vi "SimulationLoop.vi"(0 "connection ID":refnum<k5>, 7 "Cluster":T1, 11 "error in (no error)":errorcluster, 12 "Stop Simulation":bool, 13 "filter":bool=TRUE caption="Filter") -> (4 "connection ID out":refnum<k5>, 6 "Velocity":cluster{"vx":dbl, "vy":dbl, "vy":dbl}, 8 "Acceleration":cluster{"ax":dbl, "ay":dbl, "az":dbl}, 10 "Speed":i32, 14 "Simulation Ended":bool, 15 "error out":errorcluster)   [LabVIEW 2019]
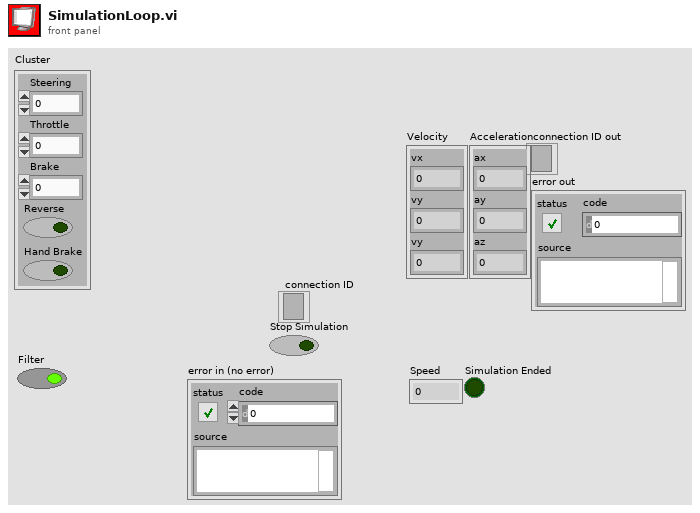
[diagram p1: front panel]
types:
  T1 = cluster{"Steering":i32, "Throttle":i32, "Brake":i32, "Reverse":bool, "Hand Brake":bool}
  T2 = cluster{"Filtered x":dbl, "Filtered x":dbl, "Filtered x":dbl}
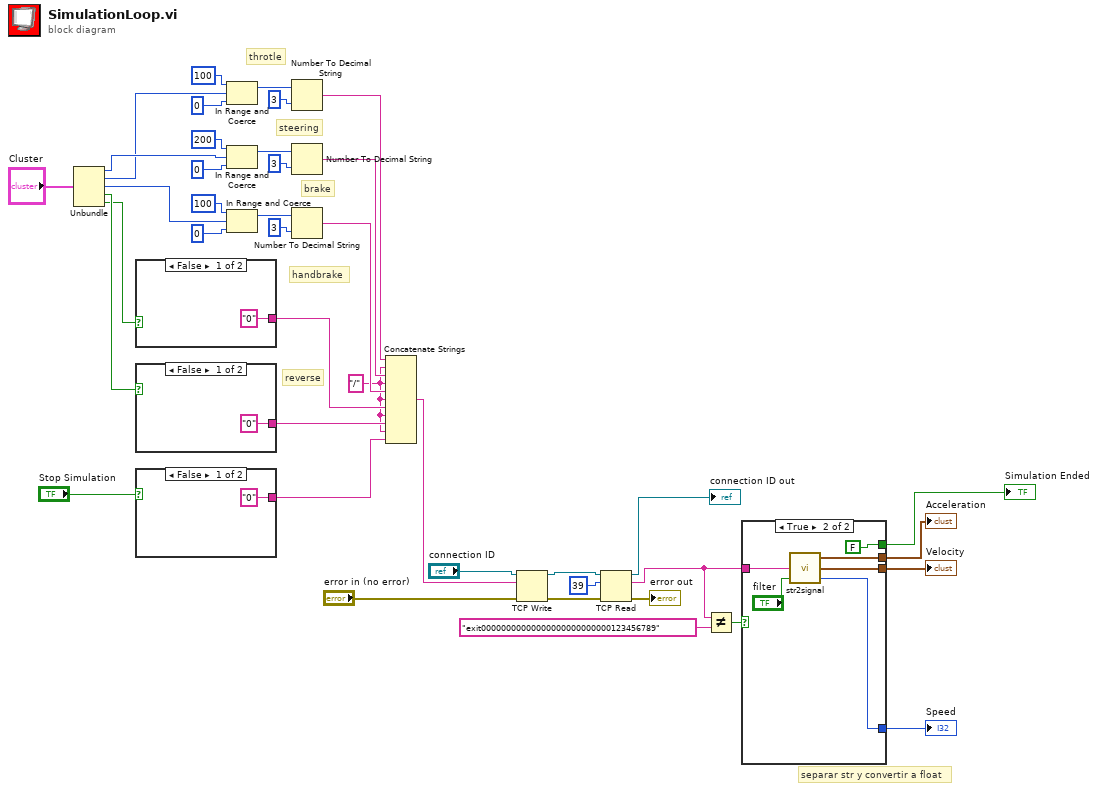
[diagram p0: block diagram]
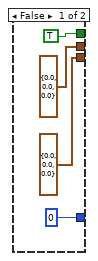
[diagram p2: hidden frame]
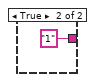
[diagram p3: hidden frame]
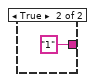
[diagram p4: hidden frame]
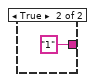
[diagram p5: hidden frame]
diagram:
  w32 = "/" ("string")
  # "reverse"
  # "handbrake"
  # "brake"
  # "steering"
  # "throtle"
  # "separar str y convertir a float"
  n1 = Unbundle("Cluster") -> ("Steering"=w5:i32, "Throttle"=w4:i32, "Brake"=w3:i32, "Reverse"=w2:bool, "Hand Brake"=w1:bool)
  n2 = case shown="False" w1 {
    tunnel: ["0" ("string") "1" ("string")] -> w34
    frame False {
    }
    frame True {
    }
  }
  n3 = case shown="False" w2 {
    tunnel: ["0" ("string") "1" ("string")] -> w33
    frame False {
    }
    frame True {
    }
  }
  n4 = case shown="False" "Stop Simulation" {
    tunnel: ["0" ("string") "1" ("string")] -> w31
    frame False {
    }
    frame True {
    }
  }
  n5 = In Range and Coerce(upper limit=100, x=w4, lower limit=0) -> (coerced(x)=w20:i32)  [unwired: 1 out]
  n6 = In Range and Coerce(upper limit=200, x=w5, lower limit=0) -> (coerced(x)=w19:i32)  [unwired: 1 out]
  n7 = In Range and Coerce(upper limit=100, x=w3, lower limit=0) -> (coerced(x)=w15:i32)  [unwired: 1 out]
  n8 = Number To Decimal String(number=w20, width (-)=i16 3) -> (decimal integer string=w38:string)
  n9 = Number To Decimal String(number=w19, width (-)=i16 3) -> (decimal integer string=w37:string)
  n10 = Number To Decimal String(number=w15, width (-)=i16 3) -> (decimal integer string=w36:string)
  n11 = Concatenate Strings(w38, w32, w37, w32, w36, w32, w34, w32, w33, w32, w31) -> (w35:string)
  n12 = TCP Write(connection ID="connection ID", data in=w35, error in (no error)="error in (no error)") -> (connection ID out=w29:refnum<k5>, error out=w28:errorcluster)  [unwired: 1 in, 1 out]
  n13 = TCP Read(connection ID=w29, bytes to read=39, error in (no error)=w28) -> (connection ID out=→"connection ID out":refnum<k5>, data out=w12:string, error out=→"error out":errorcluster)  [unwired: 2 in]
  n14 = Not Equal?(x=w12, y="exit00000000000000000000000000123456789") -> (x != y?=w13:bool)
  n15 = case shown="True" w13 {
    tunnel: [TRUE FALSE] -> w7
    tunnel: [T2 {"Filtered x"=0.0, "Filtered x"=0.0, "Filtered x"=0.0} ("Cluster 2") w56] -> w10
    tunnel: [T2 {"Filtered x"=0.0, "Filtered x"=0.0, "Filtered x"=0.0} ("Cluster") w55] -> w9
    tunnel: w12 -> [_ w54]
    tunnel: [0 ("sp") w53] -> w8
    frame False {
    }
    frame True {
      n16 = call "str2signal.vi"("filter"="filter", "srt in"=w54) -> ("sp"=w53:i32, "v"=w55:cluster{"vx":dbl, "vy":dbl, "vy":dbl}, "a"=w56:cluster{"ax":dbl, "ay":dbl, "az":dbl})  [unwired: 1 in]
    }
  }
  "Acceleration" <- w10
  "Velocity" <- w9
  "Speed" <- w8
  "Simulation Ended" <- w7
